vi "RTTERMINAL Write.vi"(8 "RTT Write":string, 11 "Down buffer index":u32) -> (0 "Return":i32)   [LabVIEW 2011, in "JLinkARM.lvlib"]
uses:
  Lib/JLinkARM.lvlib
  JLinkARM.dll
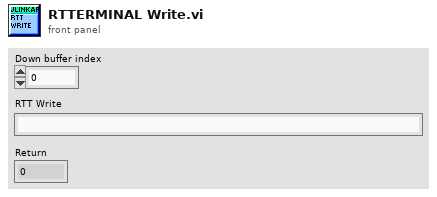
[diagram p1: front panel]
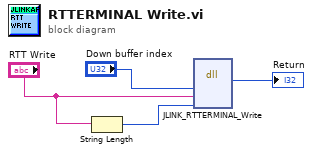
[diagram p0: block diagram]
diagram:
  n1 = String Length(string="RTT Write") -> (length=w3:i32)
  n2 = dll-call lib="C:/Documents and Settings/Anybody/Desktop/JLink_SDK_V684a/JLinkARM.dll" fn="JLINK_RTTERMINAL_Write"("BufferIndex"="Down buffer index", "sBuffer"="RTT Write", "BufferSize"=w3) -> ("return type"=→"Return":i32)  [unwired: 6 in, 2 out]
